vi "Untitled 15.vi"() -> ()   [LabVIEW 2012]
uses:
  <vilib>/Utility/NIReport.llb/NI_report.lvclass
  <vilib>/addons/database/Auxilliary.llb/DB Tools Cursor Type.ctl
  <vilib>/addons/_office/_exclsub.llb/font.ctl
  <vilib>/addons/_office/excel.llb/Excel Get Data (str).vi
  <vilib>/addons/database/Connection.llb/DB Tools Open Connec (Path).vi
  <vilib>/addons/database/Connection.llb/Conn Execute.vi
  <vilib>/addons/database/Recordset.llb/Rec Fetch Recordset Data (R).vi
  <vilib>/addons/database/Recordset.llb/Rec Destroy - Connection.vi
  <vilib>/Utility/NIReport.llb/Excel/NI_Excel.lvclass
  <vilib>/addons/_office/NI_ReportGenerationToolkit.lvlib
  <vilib>/addons/database/NI_Database_API.lvlib
panel:
  in  "start (0, 0) 4":cluster{"start row":i32, "start column":i32}
  out "error out 5":errorcluster
  out "concatenated string 2":string
  out "error out":errorcluster
  out "Numeric":i32
  in  "template (empty) 2":path=path "O:/m100schedule/Templete/MT人力配置AT機台排程.xls"
  out "concatenated string":string
  in  "start (0, 0) 3":cluster{"start row":i32, "start column":i32}
  out "ExcelRow":i32
  in  "start (0, 0)":cluster{"start row":i32, "start column":i32}
  out "x+y":i32
  out "data":string
  in  "start (0, 0) 2":cluster{"start row":i32, "start column":i32}
  out "row":i32
  in  "template (empty)":path=path "O:/m100schedule/Templete/m100-schedule temp.xls"
  out "array":string[][](array[string])
  out "error out 4":errorcluster
  out "spreadsheet string":string
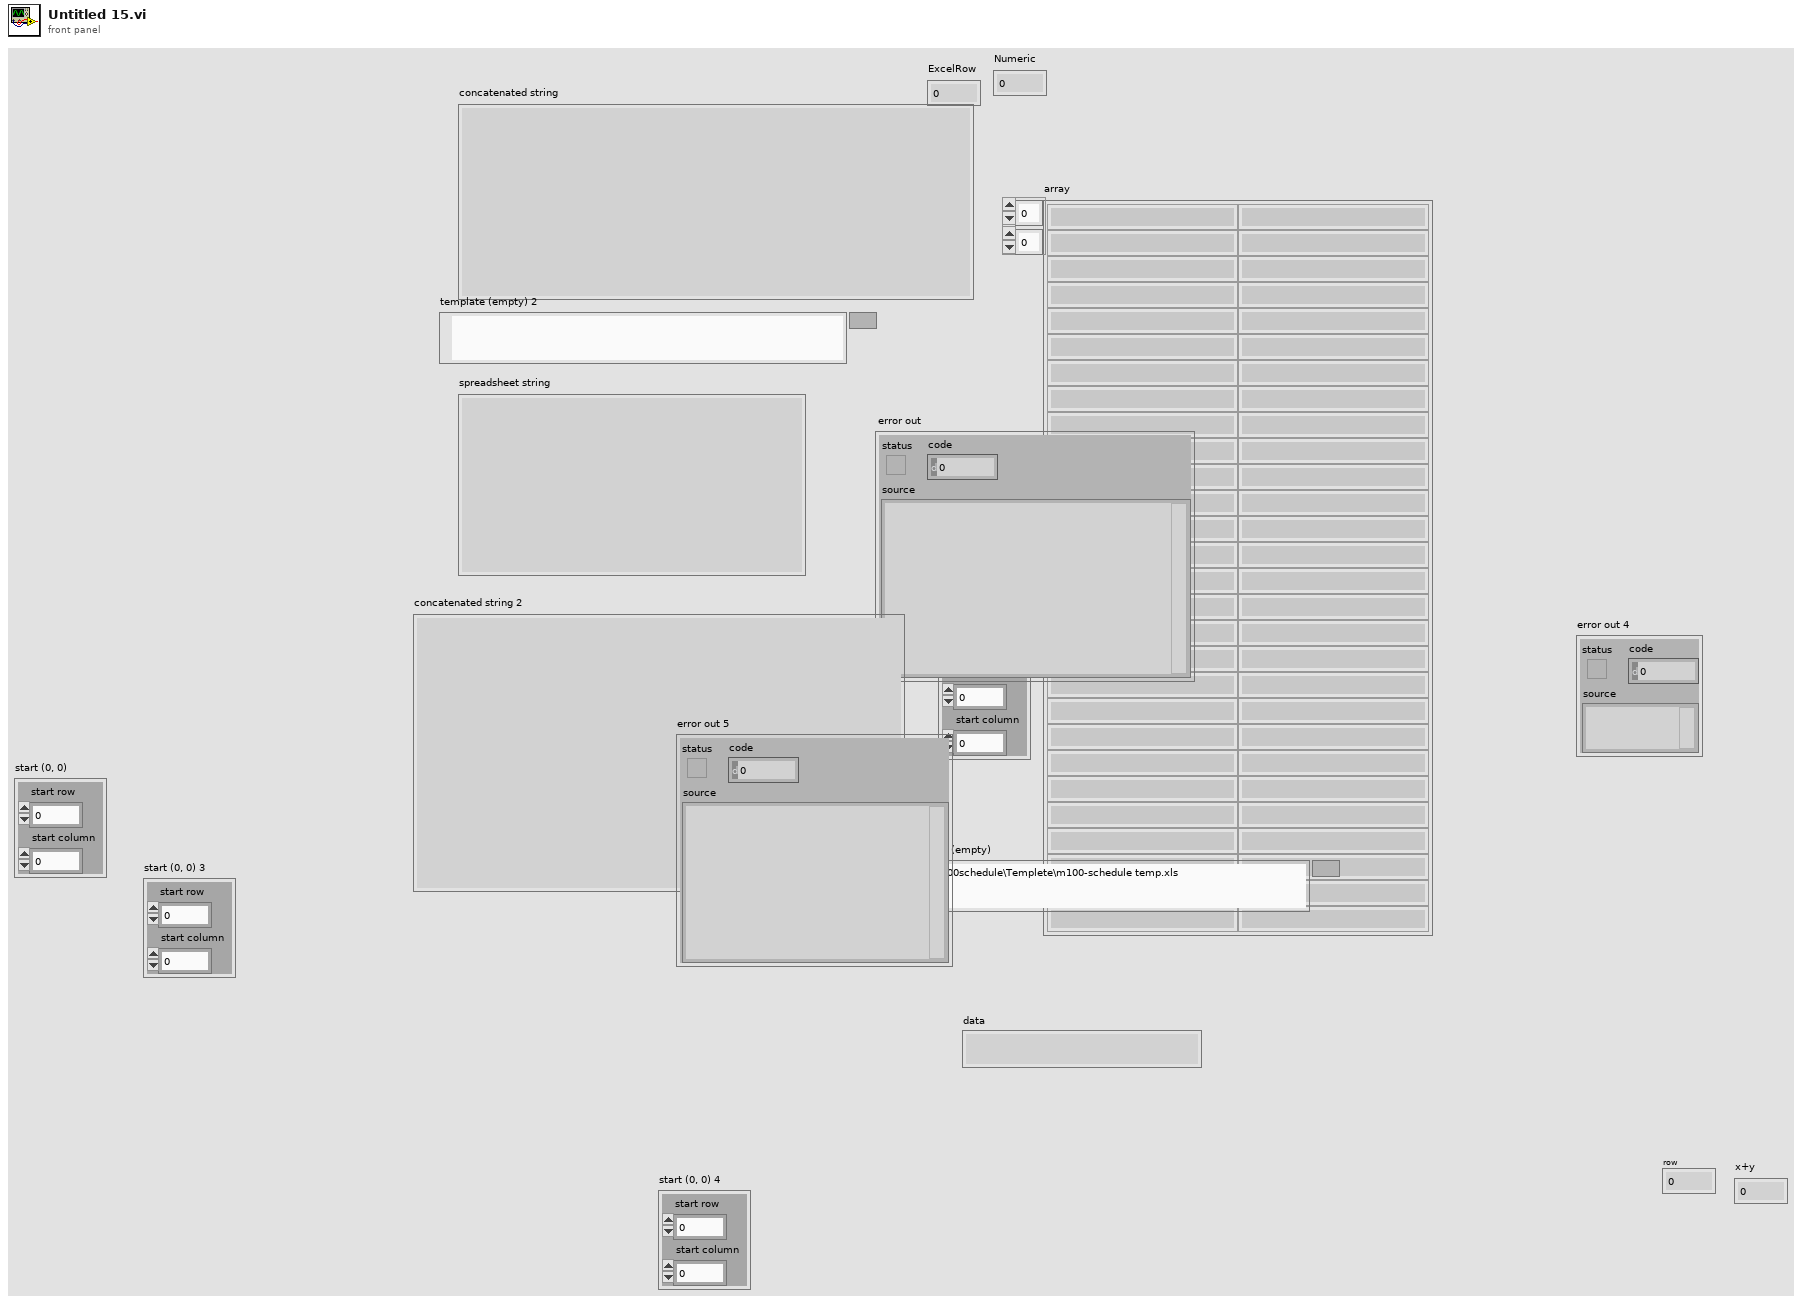
[diagram p1: front panel]
types:
  T1 = enum16{"Standard Report", "HTML", "Word", "Excel"}
  T2 = typedef "NI_ReportGenerationToolkit.lvlib/font.ctl" = cluster{"font name":string, "font size":dbl, "bold":u16, "italic":u16, "underline":u16, "strike through":u16, "font color":u32}
  T3 = cluster{"on/off":bool, "weight":i32, "color":u32}
  T4 = typedef "NI_Database_API.lvlib/DB Tools Cursor Type.ctl" = enum16{"forward-only", "keyset", "dynamic", "static"}
  T5 = typedef "NI_Database_API.lvlib/Conn ObjectReference.ctl" = refnum<k1>
  T6 = typedef "NI_Database_API.lvlib/Rec ObjectReference.ctl" = refnum<k1>
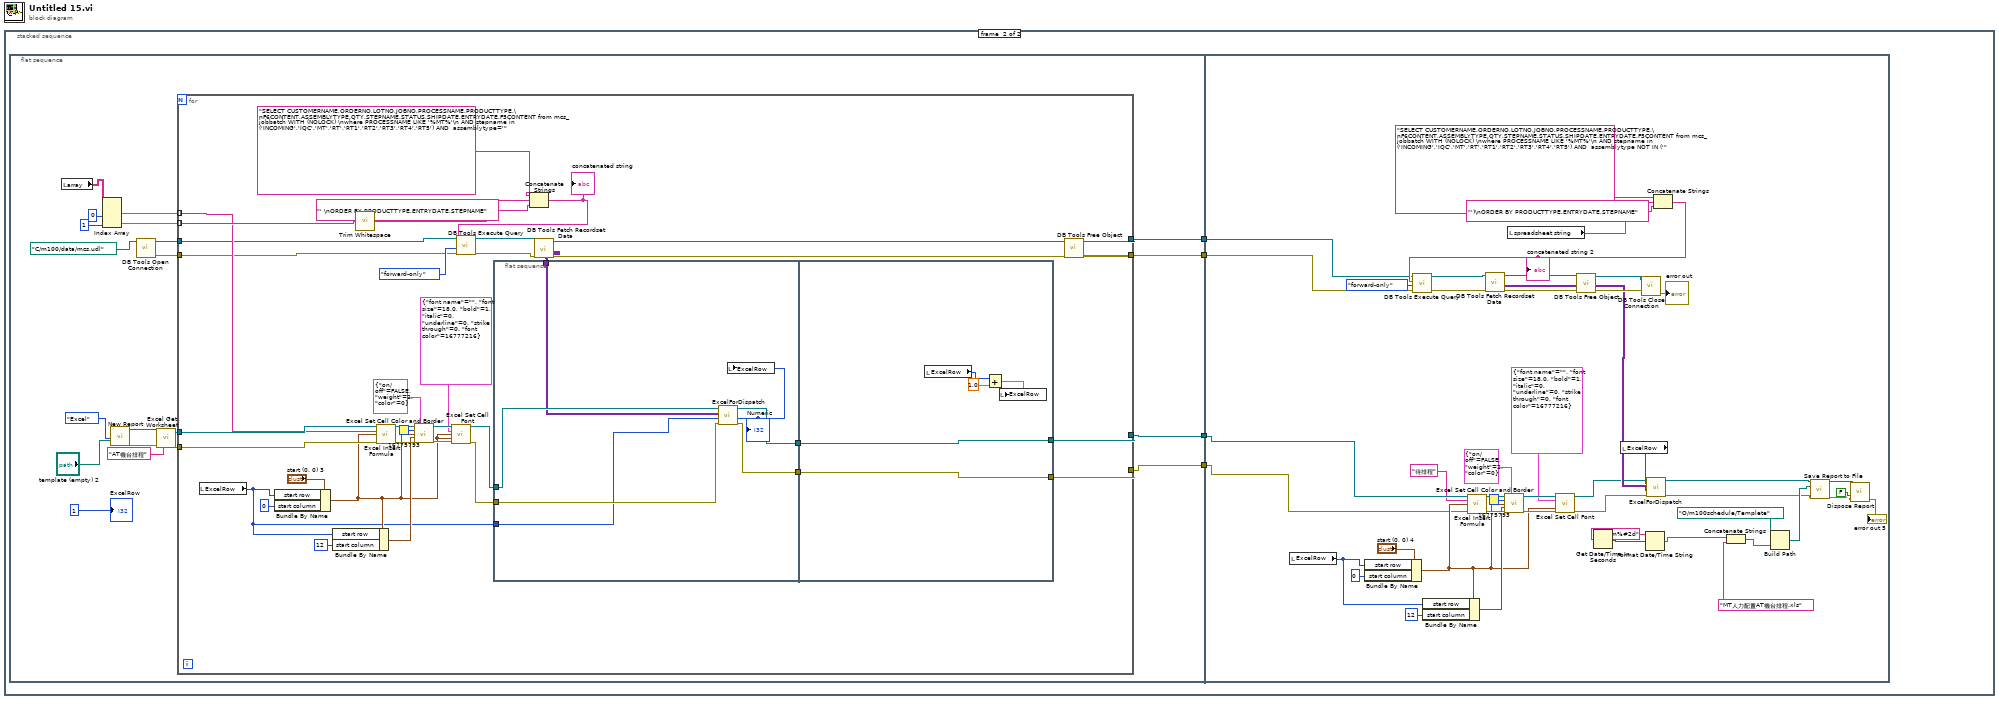
[diagram p0: block diagram]
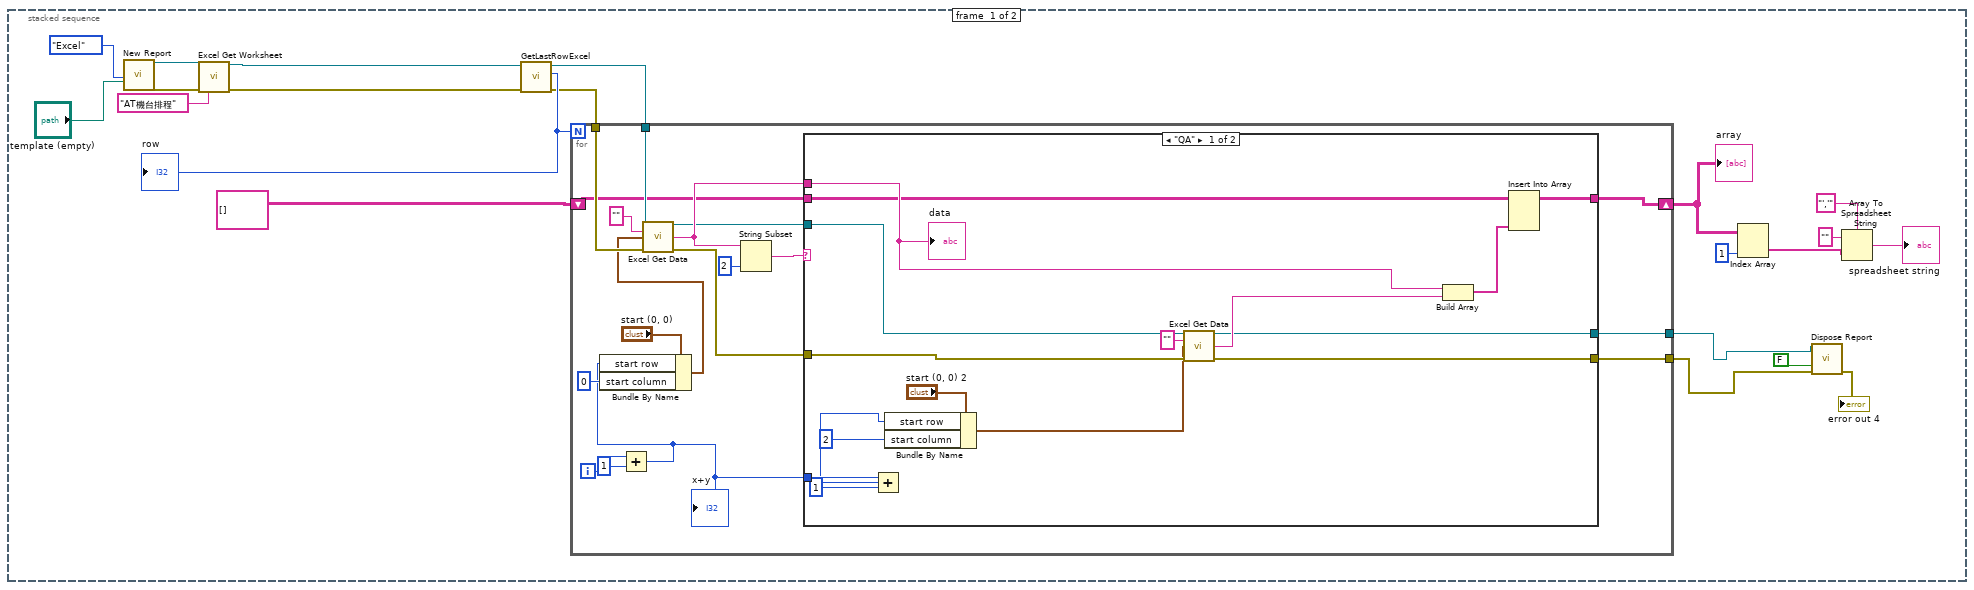
[diagram p2: hidden frame]
diagram:
  n1 = stacked-sequence {
    frame #0 {
      n2 = call <vilib>:"New Report.vi"("report type"=T1."Excel" ("Report Type"), "template (empty)"="template (empty)") -> ("report out"=w20:refnum<class "NI_report.lvclass">, "error out"=w19:errorcluster)  [unwired: 12 in]
      n3 = call <vilib>:"Excel Get Worksheet.vi"("report in"=w20, "error in (no error)"=w19, "name (\"\")"="AT機台排程" ("name (\"\")")) -> ("report out"=w18:refnum<class "NI_report.lvclass">, "error out"=w17:errorcluster)  [unwired: 11 in]
      n4 = call "GetLastRowExcel.vi"("error in (no error)"=w17, "report in"=w18) -> ("error out"=w13:errorcluster, "row"=w16:i32, "report out"=w12:refnum<class "NI_report.lvclass">)  [unwired: 7 in]
      "row" <- w16
      n5 = for {
        N: w16 -> [_]
        tunnel: w12 -> [w39]
        tunnel: w13 -> [w38]
        shift-right: [w27] -> w3
        shift-left: string[][] [] ("array") -> [w28]
        tunnel: [w23] -> w8
        tunnel: [w22] -> w7
        i -> [w34]
        n6 = Add(x=w34, y=1) -> (x+y=w24:i32)
        "x+y" <- w24
        n7 = Bundle By Name(cluster="start (0, 0)", "start row"=w24, "start column"=0) -> (w35:cluster{"start row":i32, "start column":i32})
        n8 = call-poly <vilib>:"Excel Get Data.vi"("report in"=w39, "data type"="", "start (0, 0)"=w35, "error in (no error)"=w38) -> ("report out"=w26:refnum<class "NI_report.lvclass">, "data"=w30:string, "error out"=w25:errorcluster)  [unwired: 9 in]
        n9 = String Subset(string=w30, length (rest)=2 ("length (rest)")) -> (substring=w31:string)  [unwired: 1 in]
        n10 = case shown="\"QA\"" w31 {
          tunnel: w30 -> [w55 _]
          tunnel: w28 -> [w52 w58]
          tunnel: [w53 w58] -> w27
          tunnel: w26 -> [w51 w57]
          tunnel: w25 -> [w50 w56]
          tunnel: w24 -> [w45 _]
          tunnel: [w41 w57] -> w23
          tunnel: [w40 w56] -> w22
          frame "QA" {
            n11 = Add(x=w45, y=1) -> (x+y=w43:i32)
            n12 = Bundle By Name(cluster="start (0, 0) 2", "start row"=w43, "start column"=2) -> (w48:cluster{"start row":i32, "start column":i32})
            n13 = call-poly <vilib>:"Excel Get Data.vi"("report in"=w51, "data type"="", "start (0, 0)"=w48, "error in (no error)"=w50) -> ("report out"=w41:refnum<class "NI_report.lvclass">, "data"=w42:string, "error out"=w40:errorcluster)  [unwired: 9 in]
            n14 = Build Array(w55, w42) -> (w54:string[])
            n15 = Insert Into Array(array=w52, new element=w54) -> (w53:string[][])  [unwired: 2 in]
            "data" <- w55
          }
          frame Default {
          }
        }
      }
      "array" <- w3
      n16 = Index Array(array=w3, index (col)=1 ("disabled index (col)")) -> (element=w1:string[])  [unwired: 1 in]
      n17 = call-dynamic "Dispose Report.vi"("report in"=w8, "save changes? (F)"=FALSE, "error in (no error)"=w7) -> ("error out"=→"error out 4":errorcluster)  [unwired: 12 in]
      n18 = Array To Spreadsheet String(delimiter (Tab)="','", array=w1, 3:"" ("format string")) -> (spreadsheet string=→"spreadsheet string":string)
    }
    frame #1 {
      n19 = flat-sequence {
        tunnel: [w66] -> w62
        tunnel: [w65] -> w61
        tunnel: [w64] -> w60
        tunnel: [w63] -> w59
        tunnel: w62 -> [w165]
        tunnel: w61 -> [w164]
        tunnel: w60 -> [w134]
        tunnel: w59 -> [w133]
        frame #0 {
          n20 = local read "array"() -> (w77:string[][])
          n21 = Index Array(array=w77, index (col) #1=0 ("disabled index (col)"), index (col) #2=1 ("index (col)")) -> (element #1=w76:string[], element #2=w73:string[])  [unwired: 2 in]
          n22 = call <vilib>:"New Report.vi"("report type"=T1."Excel" ("Report Type"), "template (empty)"="template (empty) 2") -> ("report out"=w81:refnum<class "NI_report.lvclass">, "error out"=w80:errorcluster)  [unwired: 12 in]
          n23 = call-poly <vilib>:"DB Tools Open Connection.vi"("connection information"=path "C:/m100/data/mcs.udl") -> ("error out"=w67:errorcluster, "connection reference"=w68:T5)  [unwired: 7 in]
          n24 = call <vilib>:"Excel Get Worksheet.vi"("report in"=w81, "error in (no error)"=w80, "name (\"\")"="AT機台排程" ("name (\"\")")) -> ("report out"=w72:refnum<class "NI_report.lvclass">, "error out"=w71:errorcluster)  [unwired: 11 in]
          n25 = for {
            tunnel: w76 -> [w106] mode=indexing
            tunnel: w73 -> [w111] mode=indexing
            tunnel: w72 -> [w108]
            tunnel: w71 -> [w107]
            tunnel: [w91] -> w64
            tunnel: [w90] -> w63
            tunnel: w68 -> [w89]
            tunnel: w67 -> [w88]
            tunnel: [w87] -> w66
            tunnel: [w86] -> w65
            n26 = local read "ExcelRow"() -> (w83:i32)
            n27 = Bundle By Name(cluster="start (0, 0) 3", "start row"=w83, "start column"=0) -> (w93:cluster{"start row":i32, "start column":i32})
            n28 = Bundle By Name(cluster=w93, "start row"=w83, "start column"=12) -> (w98:cluster{"start row":i32, "start column":i32})
            n29 = call <vilib>:"Trim Whitespace.vi"("string"=w111) -> ("trimmed string"=w110:string)  [unwired: 1 in]
            n30 = call <vilib>:"Excel Insert Formula.vi"("report in"=w108, "formula"=w106, "start (0, 0)"=w93, "error in (no error)"=w107) -> ("report out"=w103:refnum<class "NI_report.lvclass">, "error out"=w102:errorcluster)  [unwired: 10 in]
            n31 = call <vilib>:"Excel Set Cell Color and Border.vi"("report in"=w103, "inside border"=T3 {"on/off"=FALSE, "weight"=2, "color"=0}, "background color (w)"=u32 16775793, "start (-1, -1)"=w93, "end (-1, -1)"=w98, "error in (no error)"=w102) -> ("report out"=w97:refnum<class "NI_report.lvclass">, "error out"=w96:errorcluster)  [unwired: 8 in]
            n32 = call <vilib>:"Excel Set Cell Font.vi"("report in"=w97, "font"=T2 {"font name"="", "font size"=18.0, "bold"=1, "italic"=0, "underline"=0, "strike through"=0, "font color"=16777216}, "start (-1, -1)"=w93, "end (-1, -1)"=w93, "error in (no error)"=w96) -> ("report out"=w95:refnum<class "NI_report.lvclass">, "error out"=w94:errorcluster)  [unwired: 9 in]
            n33 = flat-sequence {
              tunnel: w109 -> [w124]
              tunnel: w95 -> [w126]
              tunnel: w94 -> [w125]
              tunnel: [w123] -> w85
              tunnel: [w122] -> w84
              tunnel: w83 -> [w120]
              tunnel: [w128] -> w91
              tunnel: w85 -> [w128]
              tunnel: [w127] -> w90
              tunnel: w84 -> [w127]
              frame #0 {
                n34 = call "ExcelForDispatch.vi"("error out"=w125, "RowNo"=w120, "array"=w124, "report out"=w126) -> ("error out 2"=w122:errorcluster, "Numeric"=w121:i32, "report out 2"=w123:refnum<class "NI_report.lvclass">)  [unwired: 5 in]
                "Numeric" <- w121
                n35 = local write "ExcelRow"(w121) -> ()
              }
              frame #1 {
                n36 = local read "ExcelRow"() -> (w130:i32)
                n37 = Add(x=w130, y=1.0) -> (x+y=w129:dbl)
                n38 = local write "ExcelRow"(w129) -> ()
              }
            }
            n39 = Concatenate Strings("SELECT CUSTOMERNAME,ORDERNO,LOTNO,JOBNO,PROCESSNAME,PRODUCTTYPE,\nF6CONTENT,ASSEMBLYTYPE,QTY,STEPNAME,STATUS,SHIPDATE,ENTRYDATE,F5CONTENT from mcs_jobbatch WITH (NOLOCK) \nwhere PROCESSNAME LIKE '%MT%'\n AND stepname in ('INCOMING','IQC','MT','RT','RT1','RT2','RT3','RT4','RT5') AND  assemblytype='" ("SQL query"), w110, "' \nORDER BY PRODUCTTYPE,ENTRYDATE,STEPNAME" ("string")) -> (w113:string)
            "concatenated string" <- w113
            n40 = call-poly <vilib>:"DB Tools Execute Query.vi"("error in (no error)"=w88, "cursor type"=DB_Tools_Cursor_Type."forward-only", "SQL query"=w113, "connection reference"=w89) -> ("error out"=w117:errorcluster, "recordset reference"=w119:T6)  [unwired: 4 in]
            n41 = call-poly <vilib>:"DB Tools Fetch Recordset Data.vi"("error in (no error)"=w117, "recordset reference"=w119) -> ("error out"=w116:errorcluster, "recordset data"=w109:variant[][], "recordset reference out"=w118:T6)  [unwired: 3 in]
            n42 = call-poly <vilib>:"DB Tools Free Object.vi"("error in (no error)"=w116, "recordset reference"=w118) -> ("error out"=w86:errorcluster, "connection reference"=w87:T5)  [unwired: 8 in]
          }
          "ExcelRow" <- 1
        }
        frame #1 {
          n43 = local read "ExcelRow"() -> (w137:i32)
          n44 = Bundle By Name(cluster="start (0, 0) 4", "start row"=w137, "start column"=0) -> (w139:cluster{"start row":i32, "start column":i32})
          n45 = Bundle By Name(cluster=w139, "start row"=w137, "start column"=12) -> (w142:cluster{"start row":i32, "start column":i32})
          n46 = call <vilib>:"Excel Insert Formula.vi"("report in"=w134, "formula"="待排程", "start (0, 0)"=w139, "error in (no error)"=w133) -> ("report out"=w147:refnum<class "NI_report.lvclass">, "error out"=w146:errorcluster)  [unwired: 10 in]
          n47 = call <vilib>:"Excel Set Cell Color and Border.vi"("report in"=w147, "inside border"=T3 {"on/off"=FALSE, "weight"=2, "color"=0}, "background color (w)"=u32 16775793, "start (-1, -1)"=w139, "end (-1, -1)"=w142, "error in (no error)"=w146) -> ("report out"=w141:refnum<class "NI_report.lvclass">, "error out"=w140:errorcluster)  [unwired: 8 in]
          n48 = local read "spreadsheet string"() -> (w170:string)
          n49 = call <vilib>:"Excel Set Cell Font.vi"("report in"=w141, "font"=T2 {"font name"="", "font size"=18.0, "bold"=1, "italic"=0, "underline"=0, "strike through"=0, "font color"=16777216}, "start (-1, -1)"=w139, "end (-1, -1)"=w139, "error in (no error)"=w140) -> ("report out"=w136:refnum<class "NI_report.lvclass">, "error out"=w135:errorcluster)  [unwired: 9 in]
          n50 = Get Date/Time In Seconds() -> (seconds since 1Jan1904=w152:timestamp)
          n51 = local read "ExcelRow"() -> (w166:i32)
          n52 = Format Date/Time String(time format string (%c)="%#2m%#2d", seconds (now)=w152) -> (date/time string=w150:string)  [unwired: 1 in]
          n53 = Concatenate Strings("SELECT CUSTOMERNAME,ORDERNO,LOTNO,JOBNO,PROCESSNAME,PRODUCTTYPE,\nF6CONTENT,ASSEMBLYTYPE,QTY,STEPNAME,STATUS,SHIPDATE,ENTRYDATE,F5CONTENT from mcs_jobbatch WITH (NOLOCK) \nwhere PROCESSNAME LIKE '%MT%'\n AND stepname in ('INCOMING','IQC','MT','RT','RT1','RT2','RT3','RT4','RT5') AND  assemblytype NOT IN ('" ("SQL query"), w170, "')\nORDER BY PRODUCTTYPE,ENTRYDATE,STEPNAME" ("string")) -> (w168:string)
          "concatenated string 2" <- w168
          n54 = call-poly <vilib>:"DB Tools Execute Query.vi"("error in (no error)"=w164, "cursor type"=DB_Tools_Cursor_Type."forward-only", "SQL query"=w168, "connection reference"=w165) -> ("error out"=w176:errorcluster, "recordset reference"=w178:T6)  [unwired: 4 in]
          n55 = call-poly <vilib>:"DB Tools Fetch Recordset Data.vi"("error in (no error)"=w176, "recordset reference"=w178) -> ("error out"=w175:errorcluster, "recordset data"=w167:variant[][], "recordset reference out"=w177:T6)  [unwired: 3 in]
          n56 = call-poly <vilib>:"DB Tools Free Object.vi"("error in (no error)"=w175, "recordset reference"=w177) -> ("error out"=w174:errorcluster, "connection reference"=w173:T5)  [unwired: 8 in]
          n57 = call <vilib>:"DB Tools Close Connection.vi"("error in (no error)"=w174, "connection reference"=w173) -> ("error out"=→"error out":errorcluster)  [unwired: 5 in]
          n58 = call "ExcelForDispatch.vi"("error out"=w135, "RowNo"=w166, "array"=w167, "report out"=w136) -> ("error out 2"=w154:errorcluster, "report out 2"=w155:refnum<class "NI_report.lvclass">)  [unwired: 5 in, 1 out]
          n59 = Concatenate Strings(w150, "MT人力配置AT機台排程.xls" ("string")) -> (w156:string)
          n60 = Build Path(base path=path "O:/m100schedule/Templete", name or relative path=w156) -> (appended path=w157:path)
          n61 = call-dynamic "Save Report to File.vi"("report in"=w155, "report file path"=w157, "error in (no error)"=w154) -> ("report out"=w159:refnum<class "NI_report.lvclass">, "error out"=w158:errorcluster)  [unwired: 11 in]
          n62 = call-dynamic "Dispose Report.vi"("report in"=w159, "save changes? (F)"=FALSE, "error in (no error)"=w158) -> ("error out"=→"error out 5":errorcluster)  [unwired: 12 in]
        }
      }
    }
  }
